vi "PWM_kernel.vi"(8 "Error In":errorcluster, 10 "PWM FGV Data":T1={"frequency"=5000.0, "Duty Cycle (%)"=0.0, "Axis Enum"=enum."X-axis", "Function Enum"=enum."Shutdown"} {"Duty Cycle (%)" min=0.0 max=100.0; "frequency" format="%_6g"}, 11 "Task Array in":refnum<k21>[](array[refnum])) -> (0 "Error Out":errorcluster, 3 "Task Array out":refnum<k21>[](array[refnum]))   [LabVIEW 2013]
doc: "This sub-VI provides functionality for starting, utilizing, and ending PWM tasks on the PXI controller."
uses:
  Controls/PWM_data_cluster.ctl
  Controls/table_axis_enum.ctl
  Controls/PWM_state_enum.ctl
  <vilib>/DAQmx/write.llb/DAQmx Write (Counter Frequency 1Chan 1Samp).vi
  <vilib>/DAQmx/create/channels.llb/DAQmx Create Channel (CO-Pulse Generation-Frequency).vi
  <vilib>/DAQmx/configure/timing.llb/DAQmx Timing (Implicit).vi
  <vilib>/DAQmx/miscellaneous.llb/DAQmx Fill In Error Info.vi
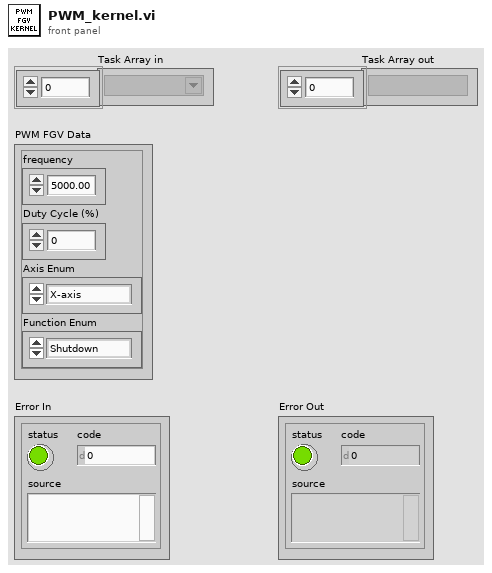
[diagram p1: front panel]
types:
  T1 = typedef "PWM_data_cluster.ctl" = cluster{"frequency":dbl, "Duty Cycle (%)":dbl, "Axis Enum":T2, "Function Enum":T3}
  T2 = typedef "table_axis_enum.ctl" = enum16{"X-axis", "Y-axis", "Z-axis", "W-axis"}
  T3 = typedef "PWM_state_enum.ctl" = enum16{"Initialize", "SetAxisSpeed", "StopAxis", "StopAll", "Shutdown"}
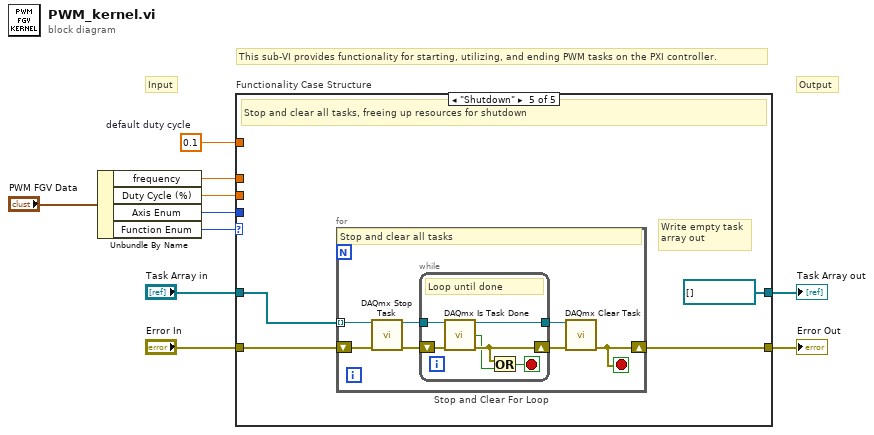
[diagram p0: block diagram]
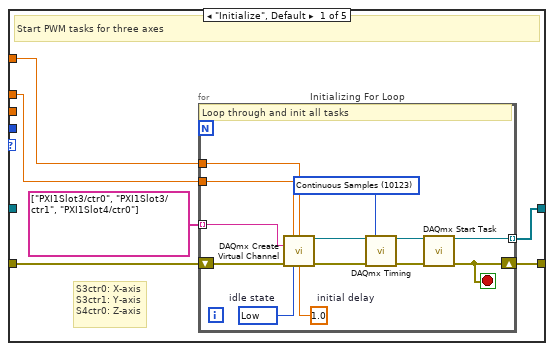
[diagram p2: hidden frame]
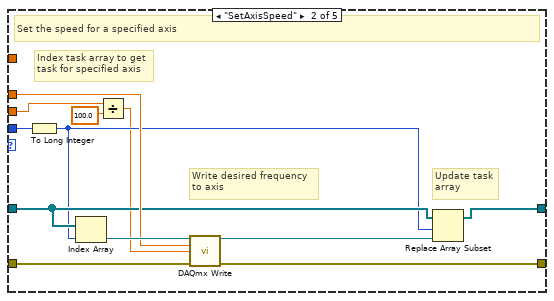
[diagram p3: hidden frame]
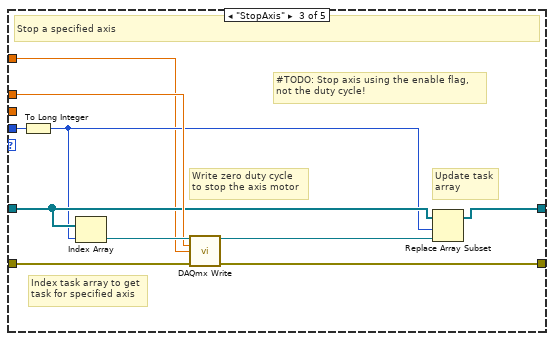
[diagram p4: hidden frame]
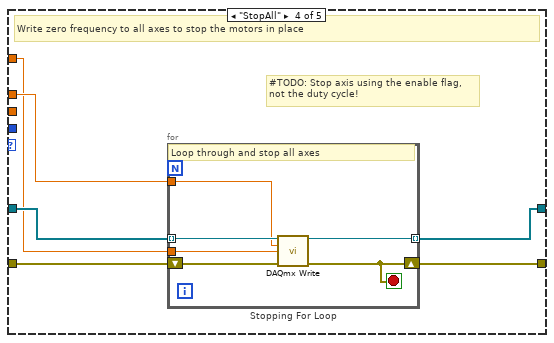
[diagram p5: hidden frame]
diagram:
  w1 = 0.1  # default duty cycle
  # "Output"
  # "Input"
  # "This sub-VI provides functionality for starting, utilizing, and ending PWM tasks on the PXI controller."
  n1 = Unbundle By Name("PWM FGV Data") -> ("frequency"=w2:dbl, "Duty Cycle (%)"=w3:dbl, "Axis Enum"=w4:T2, "Function Enum"=w5:T3)
  n2 = case "Functionality Case Structure" shown="\"Shutdown\"" w5 {
    tunnel: "Error In" -> [w16 w40 w51 w55 w66]
    tunnel: [w15 w38 w50 w57 w65] -> w9
    tunnel: [w13 w34 w43 w56 refnum<k21>[] []] -> w8
    tunnel: "Task Array in" -> [_ w35 w46 w54 w67]
    tunnel: w4 -> [_ w41 w49 _ _]
    tunnel: w3 -> [_ w32 _ _ _]
    tunnel: w2 -> [w12 w37 w47 w53 _]
    tunnel: w1 -> [w11 _ w42 w52 _]
    frame "Initialize", Default {
      # "S3ctr0: X-axis\nS3ctr1: Y-axis\nS4ctr0: Z-axis"
      # "Start PWM tasks for three axes"
      n3 = for "Initializing For Loop" {
        shift-right: [w18] -> w15
        shift-left: w16 -> [w29]
        tunnel: tag[] ["PXI1Slot3/ctr0", "PXI1Slot3/ctr1", "PXI1Slot4/ctr0"] -> [w27] mode=indexing
        tunnel: [w20] -> w13 mode=indexing
        tunnel: w12 -> [w23]
        tunnel: w11 -> [w17]
        stop <- w18 stop-if-true
        w21 = 10214 items=["High"=10192, "Low"=10214]  # idle state
        w22 = 1.0  # initial delay
        w25 = 10123 items=["Finite Samples"=10178, "Continuous Samples"=10123, "Hardware Timed Single Point"=12522] ("sample mode")
        # "Loop through and init all tasks"
        n4 = call-poly <vilib>:"DAQmx Create Virtual Channel.vi"("frequency"=w23, "duty cycle"=w17, "counter"=w27, "error in"=w29, "idle state"=w21, "initial delay"=w22) -> ("task out"=w26:refnum<k21>, "error out"=w28:errorcluster)  [unwired: 8 in]
        n5 = call-poly <vilib>:"DAQmx Timing.vi"("task/channels in"=w26, "sample mode"=w25, "error in"=w28) -> ("task out"=w24:refnum<k21>, "error out"=w19:errorcluster)  [unwired: 11 in]
        n6 = call <vilib>:"DAQmx Start Task.vi"("task/channels in"=w24, "error in"=w19) -> ("task out"=w20:refnum<k21>, "error out"=w18:errorcluster)  [unwired: 12 in]
      }
    }
    frame "SetAxisSpeed" {
      # "Update task\narray"
      # "Write desired frequency\nto axis"
      # "Index task array to get\ntask for specified axis"
      # "Set the speed for a specified axis"
      n7 = To Long Integer(number=w41) -> (32bit integer=w33:i32)
      n8 = Index Array(array=w35, index=w33) -> (element=w39:refnum<k21>)
      n9 = Divide(x=w32, y=100.0) -> (x/y=w31:dbl)
      n10 = call-poly <vilib>:"DAQmx Write.vi"("task/channels in"=w39, "frequency"=w37, "duty cycle"=w31, "error in"=w40) -> ("task out"=w36:refnum<k21>, "error out"=w38:errorcluster)  [unwired: 9 in, 1 out]
      n11 = Replace Array Subset(array=w35, new element=w36, index=w33) -> (w34:refnum<k21>[])
    }
    frame "StopAxis" {
      # "Update task\narray"
      # "Index task array to get\ntask for specified axis"
      # "#TODO: Stop axis using the enable flag,\nnot the duty cycle!"
      # "Write zero duty cycle\nto stop the axis motor"
      # "Stop a specified axis"
      n12 = To Long Integer(number=w49) -> (32bit integer=w45:i32)
      n13 = Index Array(array=w46, index=w45) -> (element=w48:refnum<k21>)
      n14 = call-poly <vilib>:"DAQmx Write.vi"("task/channels in"=w48, "frequency"=w47, "duty cycle"=w42, "error in"=w51) -> ("task out"=w44:refnum<k21>, "error out"=w50:errorcluster)  [unwired: 9 in, 1 out]
      n15 = Replace Array Subset(array=w46, new element=w44, index=w45) -> (w43:refnum<k21>[])
    }
    frame "StopAll" {
      # "#TODO: Stop axis using the enable flag,\nnot the duty cycle!"
      # "Write zero frequency to all axes to stop the motors in place"
      n16 = for "Stopping For Loop" {
        shift-right: [w60] -> w57
        shift-left: w55 -> [w63]
        tunnel: [w61] -> w56 mode=indexing
        tunnel: w54 -> [w62] mode=indexing
        tunnel: w53 -> [w59]
        tunnel: w52 -> [w58]
        stop <- w60 stop-if-true
        # "Loop through and stop all axes"
        n17 = call-poly <vilib>:"DAQmx Write.vi"("task/channels in"=w62, "frequency"=w59, "duty cycle"=w58, "error in"=w63) -> ("task out"=w61:refnum<k21>, "error out"=w60:errorcluster)  [unwired: 9 in, 1 out]
      }
    }
    frame "Shutdown" {
      # "Write empty task\narray out"
      # "Stop and clear all tasks, freeing up resources for shutdown"
      n18 = for "Stop and Clear For Loop" {
        shift-right: [w74] -> w65
        shift-left: w66 -> [w68]
        tunnel: w67 -> [w69] mode=indexing
        stop <- w74 stop-if-true
        # "Stop and clear all tasks"
        n19 = call <vilib>:"DAQmx Stop Task.vi"("task/channels in"=w69, "error in"=w68) -> ("task out"=w72:refnum<k21>, "error out"=w73:errorcluster)  [unwired: 12 in]
        n20 = while {
          tunnel: [w80] -> w71
          tunnel: w72 -> [w78]
          shift-right: [w76] -> w70
          shift-left: w73 -> [w79]
          stop <- w77 stop-if-true
          # "Loop until done"
          n21 = call <vilib>:"DAQmx Is Task Done.vi"("task/channels in"=w78, "error in"=w79) -> ("task out"=w80:refnum<k21>, "task done?"=w75:bool, "error out"=w76:errorcluster)  [unwired: 11 in]
          n22 = Or(x=w76, y=w75) -> (x .or. y?=w77:bool)
        }
        n23 = call <vilib>:"DAQmx Clear Task.vi"("task in"=w71, "error in"=w70) -> ("error out"=w74:errorcluster)  [unwired: 13 in]
      }
    }
  }
  "Error Out" <- w9
  "Task Array out" <- w8
